vi "Actor Core.vi"(8 "error in":errorcluster, 11 "Child_1 in":refnum<class "GUI_Class.lvclass">) -> (0 "error out":errorcluster, 3 "Actor out":refnum<class "Actor.lvclass">)   [LabVIEW 2023, in "GUI_Actor.lvlib" / "GUI_Class.lvclass"]
doc: "(<B>Filename</B>: Actor Framework.lvlib:Actor.lvclass:Actor Core.vi)\n\nReceives messages to the actor, reacts to them, and initiates any error handling that may shut the actor down.\n\nDescendant classes may override this VI to append parallel tasks for the actor to complete while it handles messages. Overrides use the Call Parent Class Method node."
uses:
  GUI_Class.lvclass
  <vilib>/ActorFramework/Actor/Actor.lvclass
  GUI_Class.lvclass/GUI_Class.ctl
  Abstraction_Interface_Class/Abstraction_Interface_Class.lvclass
panel:
  out "Random Number":dbl
  out "Actor_Name":string
  in  "Console":string
  # "GUI"
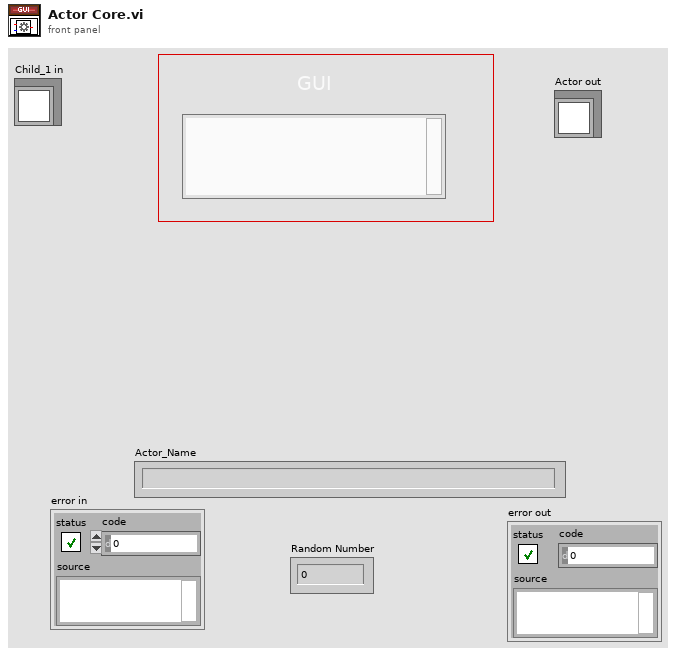
[diagram p1: front panel]
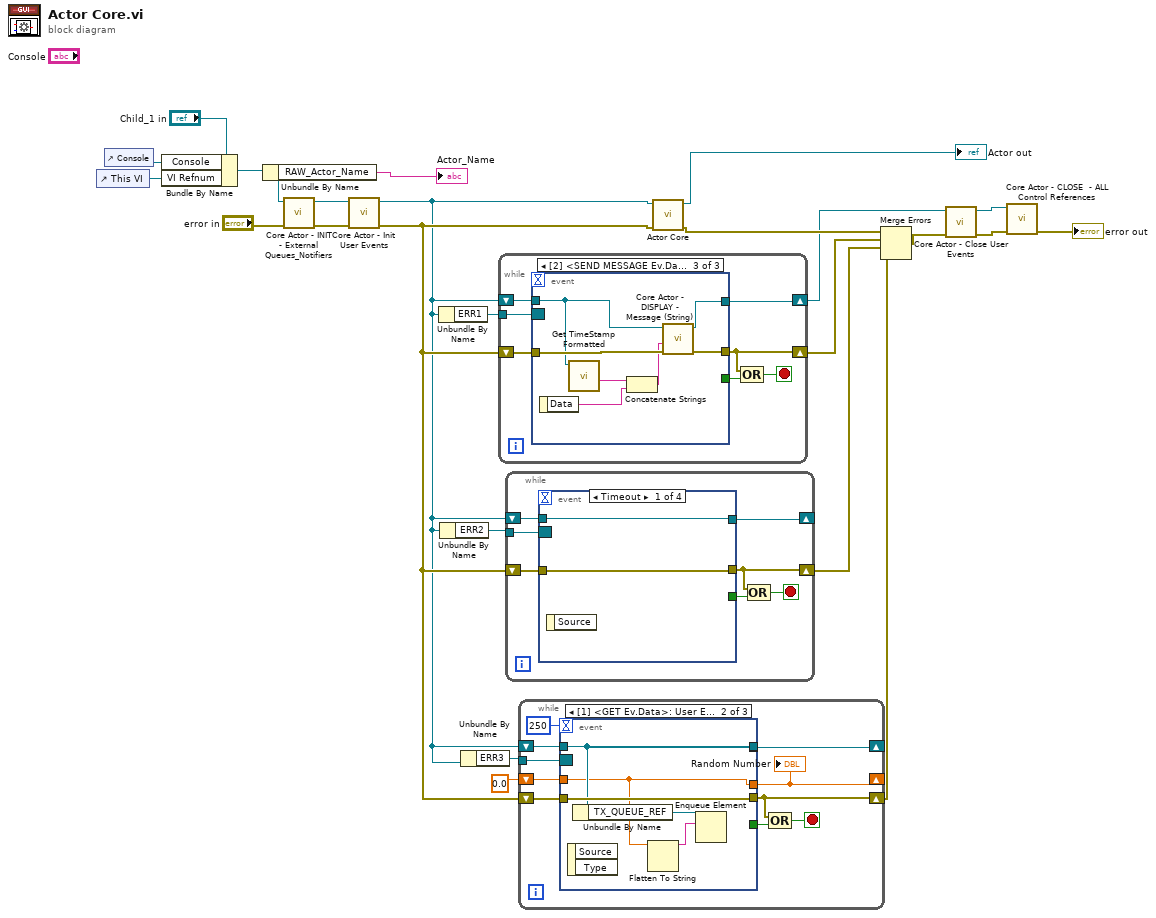
[diagram p0: block diagram]
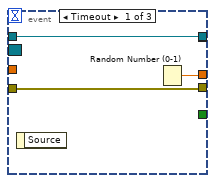
[diagram p2: hidden frame]
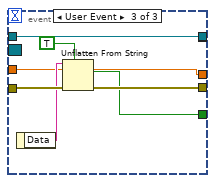
[diagram p3: hidden frame]
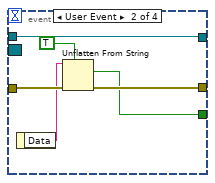
[diagram p4: hidden frame]
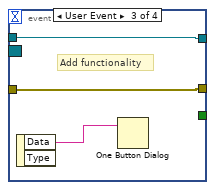
[diagram p5: hidden frame]
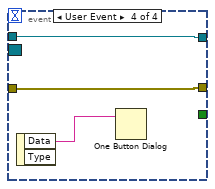
[diagram p6: hidden frame]
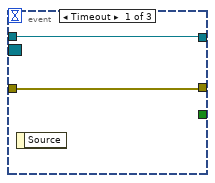
[diagram p7: hidden frame]
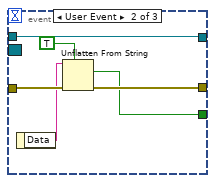
[diagram p8: hidden frame]
diagram:
  n1 = control-ref of="This VI"() -> (w17:refnum<vi>)
  n2 = control-ref of="Console"() -> (w18:refnum<vi>)
  n3 = Bundle By Name(cluster="Child_1 in", "Console"=w18, "VI Refnum"=w17) -> (w7:refnum<class "GUI_Class.lvclass">)
  n4 = Unbundle By Name(w7) -> ("RAW_Actor_Name"=→"Actor_Name":string)
  n5 = call-dynamic "Core Actor - INIT - External Queues_Notifiers.vi"("error in (no error)"="error in", "Child_1_Class in"=w7) -> ("error out"=w22:errorcluster, "Child_1_Class out"=w21:refnum<class "GUI_Class.lvclass">)  [unwired: 8 in]
  n6 = call-dynamic "Core Actor - Init User Events.vi"("error in (no error)"=w22, "Child_1_Class in"=w21) -> ("error out"=w4:errorcluster, "Child_1_Class out"=w3:refnum<class "GUI_Class.lvclass">)  [unwired: 8 in]
  n7 = Unbundle By Name(w3) -> ("ERR1"=w13:refnum<event-registration>)
  n8 = Unbundle By Name(w3) -> ("ERR2"=w9:refnum<event-registration>)
  n9 = Unbundle By Name(w3) -> ("ERR3"=w5:refnum<event-registration>)
  n10 = while {
    shift-right: [w27] -> w10
    shift-left: w4 -> [w29]
    shift-right: [w30] -> w12
    shift-left: w3 -> [w31]
    tunnel: w13 -> [w28]
    stop <- w25 stop-if-true
    n11 = event shown="[2] <SEND MESSAGE Ev.Data>: User Event" {
      selector: w28 -> [_ _ _]
      dyn-events: _ -> [_ _ _]
      timeout: _ -> [_ _ _]
      tunnel: w31 -> [w33 w34 w43]
      tunnel: [w33 w34 w44] -> w30
      tunnel: w29 -> [w32 w39 w46]
      tunnel: [w32 w36 w45] -> w27
      tunnel: [_ w35 _] -> w26
      event Timeout {
        n12 = event-data() -> ()  [unwired: 1 in, 1 out]
      }
      event User Event {
        n13 = event-data() -> ("Data"=w38:string)  [unwired: 1 in]
        n14 = Unflatten From String(type=TRUE, binary string=w38, error in (no error)=w39) -> (value=w35:bool, error out=w36:errorcluster)  [unwired: 2 in, 1 out]
      }
      event User Event {
        n15 = event-data() -> ("Data"=w41:string)  [unwired: 1 in]
        n16 = call-dynamic "Get TimeStamp Formatted.vi"("Child_1 in"=w43) -> ("TimeStamp Formatted"=w42:string)  [unwired: 8 in, 2 out]
        n17 = Concatenate Strings(w42, w41) -> (w40:string)
        n18 = call-dynamic "Core Actor - DISPLAY - Message (String).vi"("error in (no error)"=w46, "Value"=w40, "Child_1_Class in"=w43) -> ("error out"=w45:errorcluster, "Child_1_Class out"=w44:refnum<class "GUI_Class.lvclass">)  [unwired: 7 in]
      }
    }
    n19 = Compound Arithmetic op=OR(w27, w26) -> (w25:bool)
  }
  n20 = while {
    shift-right: [w49] -> w8
    shift-left: w4 -> [w51]
    shift-right: [w52] -> _
    shift-left: w3 -> [w53]
    tunnel: w9 -> [w50]
    stop <- w47 stop-if-true
    n21 = event shown="[0] Timeout" {
      selector: w50 -> [_ _ _ _]
      dyn-events: _ -> [_ _ _ _]
      timeout: _ -> [_ _ _ _]
      tunnel: w53 -> [w55 w56 w64 w66]
      tunnel: [w55 w56 w64 w66] -> w52
      tunnel: w51 -> [w54 w61 w63 w67]
      tunnel: [w54 w58 w63 w67] -> w49
      tunnel: [_ w57 _ _] -> w48
      event Timeout {
        n22 = event-data() -> ()  [unwired: 1 in, 1 out]
      }
      event User Event {
        n23 = event-data() -> ("Data"=w60:string)  [unwired: 1 in]
        n24 = Unflatten From String(type=TRUE, binary string=w60, error in (no error)=w61) -> (value=w57:bool, error out=w58:errorcluster)  [unwired: 2 in, 1 out]
      }
      event User Event {
        # "Add functionality"
        n25 = event-data() -> ("Data"=w62:string)  [unwired: 1 in, 1 out]
        n26 = One Button Dialog(message=w62) -> ()  [unwired: 1 in, 1 out]
      }
      event User Event {
        n27 = event-data() -> ("Data"=w65:string)  [unwired: 1 in, 1 out]
        n28 = One Button Dialog(message=w65) -> ()  [unwired: 1 in, 1 out]
      }
    }
    n29 = Compound Arithmetic op=OR(w49, w48) -> (w47:bool)
  }
  n30 = while {
    shift-right: [w73] -> w2
    shift-left: w4 -> [w75]
    shift-right: [w76] -> _
    shift-left: w3 -> [w77]
    tunnel: w5 -> [w74]
    shift-right: [w68] -> _
    shift-left: 0.0 -> [w69]
    stop <- w71 stop-if-true
    n31 = event shown="[1] <GET Ev.Data>: User Event" {
      selector: w74 -> [_ _ _]
      dyn-events: _ -> [_ _ _]
      timeout: 250 -> [_ _ _]
      tunnel: w77 -> [w80 w84 w87]
      tunnel: [w80 w84 w87] -> w76
      tunnel: w75 -> [w79 w85 w92]
      tunnel: [w79 w85 w89] -> w73
      tunnel: [_ _ w88] -> w72
      tunnel: w69 -> [_ w81 w86]
      tunnel: [w78 w81 w86] -> w68
      tunnel: [_ w84 _] -> _
      event Timeout {
        n32 = event-data() -> ()  [unwired: 1 in, 1 out]
        n33 = Random Number (0-1)() -> (number: 0 to 1=w78:dbl)
      }
      event User Event {
        n34 = event-data() -> ()  [unwired: 1 in, 2 out]
        n35 = Unbundle By Name(w84) -> ("TX_QUEUE_REF"=w83:refnum<queue>)
        n36 = Flatten To String(anything=w81) -> (data string=w82:string)  [unwired: 3 in, 2 out]
        n37 = Enqueue Element(queue=w83, element=w82) -> ()  [unwired: 2 in, 3 out]
      }
      event User Event {
        n38 = event-data() -> ("Data"=w91:string)  [unwired: 1 in]
        n39 = Unflatten From String(type=TRUE, binary string=w91, error in (no error)=w92) -> (value=w88:bool, error out=w89:errorcluster)  [unwired: 2 in, 1 out]
      }
    }
    "Random Number" <- w68
    n40 = Compound Arithmetic op=OR(w73, w72) -> (w71:bool)
  }
  n41 = call-parent "Actor Core.vi"("error in"=w4, "Actor in"=w3) -> ("error out"=w20:errorcluster, "Actor out"=→"Actor out":refnum<class "Actor.lvclass">)  [unwired: 8 in]
  n42 = Merge Errors(w20, w10, w8, w2) -> (w11:errorcluster)
  n43 = call-dynamic "Core Actor - Close User Events.vi"("error in (no error)"=w11, "Child_1_Class in"=w12) -> ("error out"=w16:errorcluster, "Child_1_Class out"=w14:refnum<class "GUI_Class.lvclass">)  [unwired: 8 in]
  n44 = call-dynamic "Core Actor - CLOSE  - ALL Control References.vi"("error in (no error)"=w16, "Child_1_Class in"=w14) -> ("error out"=→"error out":errorcluster)  [unwired: 8 in, 1 out]
